vi "MovePos3.vi"(7 "In Contact in":bool, 10 "Position 3":bool, 11 "UiDefinition 2":T1) -> (3 "In Contact out":bool)   [LabVIEW 2020]
uses:
  UIReferences.ctl
  D:/LabviewDXFViewer/LabviewDXFViewer/bin/Release/LabviewDXFViewer.exe
  LabviewDXFViewer/bin/Release/LabviewDXFViewer.exe
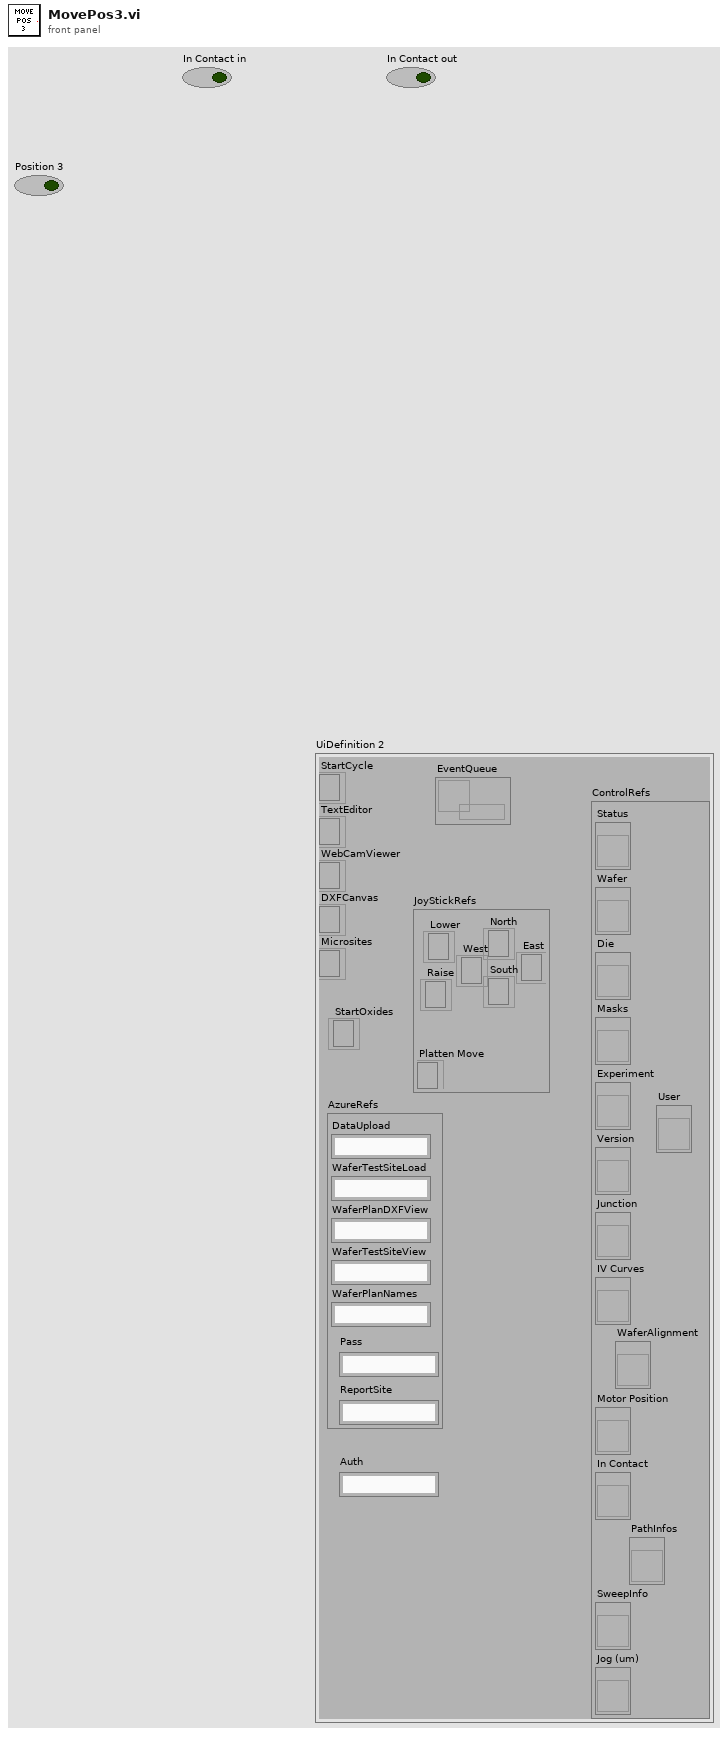
[diagram p1: front panel]
types:
  T1 = typedef "UIReferences.ctl" = cluster{"StartCycle":refnum<k24>, "TextEditor":refnum<k24>, "WebCamViewer":refnum<k24>, "DXFCanvas":refnum<k24>, "Microsites":refnum<k24>, "JoyStickRefs":cluster{"North":refnum<k24>, "Lower":refnum<k24>, "Raise":refnum<k24>, "Platten Move":refnum<k24>, "West":refnum<k24>, "East":refnum<k24>, "South":refnum<k24>}, "AzureRefs":cluster{"DataUpload":string, "WaferTestSiteLoad":string, "WaferPlanDXFView":string, "WaferTestSiteView":string, "WaferPlanNames":string, "Pass":string, "ReportSite":string}, "ControlRefs":cluster{"Status":refnum<vi>, "Wafer":refnum<vi>, "Die":refnum<vi>, "Masks":refnum<vi>, "Experiment":refnum<vi>, "Version":refnum<vi>, "Junction":refnum<vi>, "IV Curves":refnum<vi>, "Motor Position":refnum<vi>, "In Contact":refnum<vi>, "SweepInfo":refnum<vi>, "Jog (um)":refnum<vi>, "PathInfos":refnum<vi>, "User":refnum<vi>, "WaferAlignment":refnum<vi>}, "EventQueue":refnum<queue>, "StartOxides":refnum<k24>, "Auth":string}
  T2 = typedef "WaferAlignmentType.ctl" = cluster{"Wafer Units to microns":dbl, "Rotation Misalign":dbl[], "Scale Misalign":dbl, "Steps Per micron":dbl, "Position 1":i32[], "Position 2":i32[], "Lift Distance":i32, "Position 3":i32[], "Jog Height":i32}
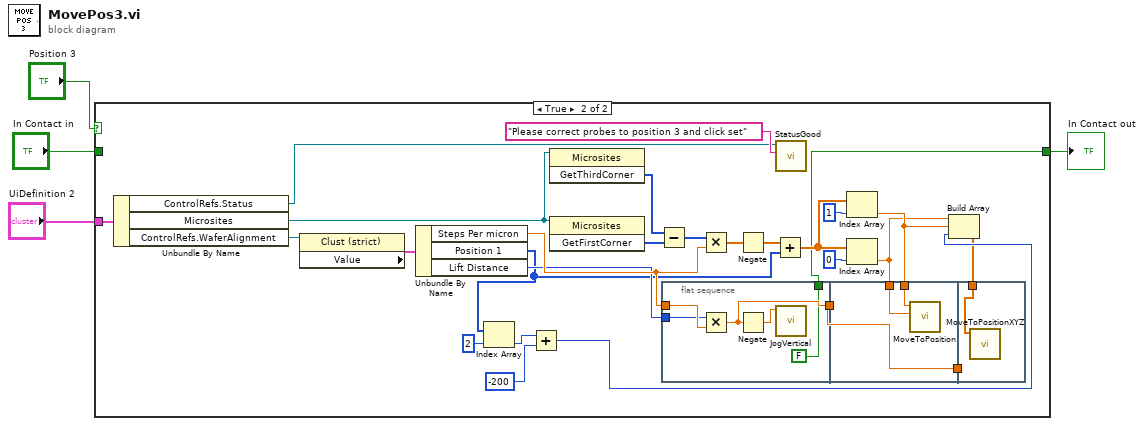
[diagram p0: block diagram]
diagram:
  n1 = case shown="True" "Position 3" {
    tunnel: [w5 w19] -> w3
    tunnel: "In Contact in" -> [w5 _]
    tunnel: "UiDefinition 2" -> [_ w16]
    frame False {
    }
    frame True {
      n2 = Unbundle By Name(w16) -> ("ControlRefs.Status"=w14:refnum<vi>, "Microsites"=w15:refnum<k24>, "ControlRefs.WaferAlignment"=w18:refnum<vi>)
      n3 = property class="Clust (strict)"(reference=w18) -> ("Value"=w17:T2)  [unwired: 1 in, 2 out]
      n4 = Unbundle By Name(w17) -> ("Steps Per micron"=w21:dbl, "Position 1"=w10:i32[], "Lift Distance"=w20:i32)
      n5 = Index Array(array=w10, index=2) -> (element=w12:i32)
      n6 = Add(x=w12, y=-200) -> (x+y=w7:i32)
      n7 = invoke class="Microsites" method="GetThirdCorner"(reference=w15) -> ("GetThirdCorner"=w32:i32[])  [unwired: 2 in, 2 out]
      n8 = invoke class="Microsites" method="GetFirstCorner"(reference=w15) -> ("GetFirstCorner"=w30:i32[])  [unwired: 2 in, 2 out]
      n9 = Subtract(x=w32, y=w30) -> (x-y=w31:i32[])
      n10 = flat-sequence {
        tunnel: w21 -> [w36]
        tunnel: [w35] -> w27
        tunnel: w20 -> [w34]
        tunnel: [FALSE ("In Contact")] -> w19
        tunnel: w8 -> [w40]
        tunnel: w9 -> [w39]
        tunnel: [w38] -> w28
        tunnel: w27 -> [w38]
        tunnel: w28 -> [_]
        tunnel: w6 -> [w41]
        frame #0 {
          n11 = Multiply(x=w34, y=w36) -> (x*y=w35:dbl)
          n12 = Negate(x=w35) -> (-x=w37:dbl)
          n13 = call "JogVertical.vi"("Numeric"=w37) -> ()  [unwired: 11 in]
        }
        frame #1 {
          n14 = call "MoveToPosition.vi"("Y"=w40, "X"=w39) -> ()  [unwired: 10 in]
        }
        frame #2 {
          n15 = call "MoveToPositionXYZ.vi"("Array"=w41) -> ()  [unwired: 11 in]
        }
      }
      n16 = Multiply(x=w31, y=w21) -> (x*y=w29:dbl[])
      n17 = Negate(x=w29) -> (-x=w23:dbl[])
      n18 = Add(x=w23, y=w10) -> (x+y=w24:dbl[])
      n19 = call "StatusGood.vi"("Text.Text"="Please correct probes to position 3 and click set" ("Status"), "String in"=w14) -> ()  [unwired: 10 in]
      n20 = Index Array(array=w24, index=1) -> (element=w9:dbl)
      n21 = Index Array(array=w24, index=0) -> (element=w8:dbl)
      n22 = Build Array(w8, w9, w7) -> (w6:dbl[])
    }
  }
  "In Contact out" <- w3
